vi "配置数据迁移.vi"(8 "error in (no error)":errorcluster) -> (0 "error out":errorcluster)   [LabVIEW 2016]
uses:
  <vilib>/Utility/config.llb/Read Key (String).vi
  <vilib>/Utility/config.llb/Write Key (String).vi
  <vilib>/Utility/config.llb/NI_LVConfig.lvlib
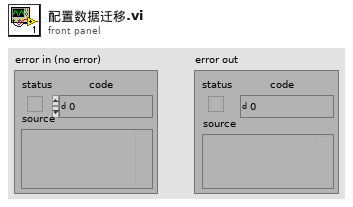
[diagram p1: front panel]
types:
  T1 = typedef "NI_LVConfig.lvlib/Config Data RefNum.ctl" = refnum<k1>
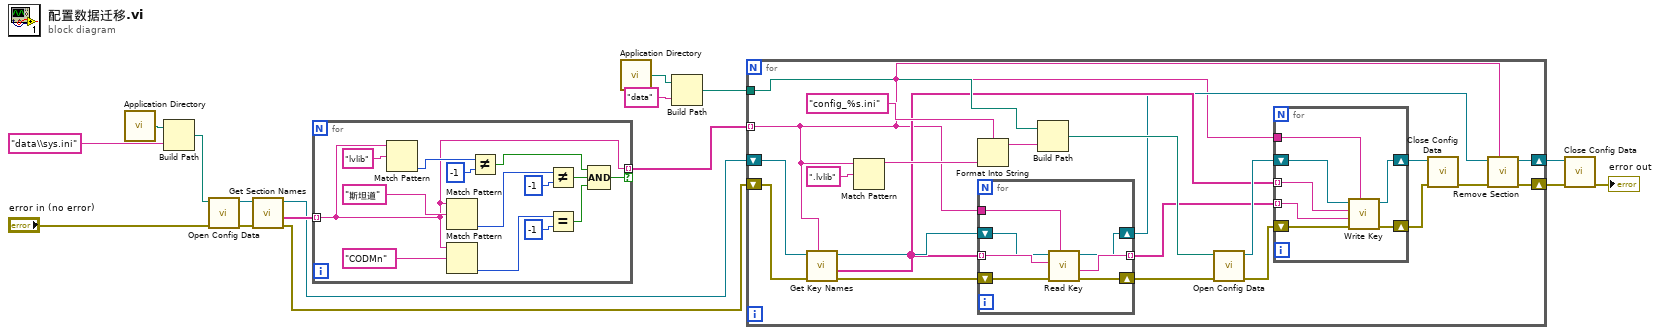
[diagram p0: block diagram]
diagram:
  n1 = call <vilib>:"Application Directory.vi"() -> ("Application Directory"=w14:path)
  n2 = Build Path(base path=w14, name or relative path="data\\sys.ini" ("名称或相对路径")) -> (appended path=w16:path)
  n3 = call <vilib>:"Open Config Data.vi"("error in (no error)"="error in (no error)", "configuration file path"=w16) -> ("error out"=w13:errorcluster, "refnum"=w12:T1)  [unwired: 7 in, 1 out]
  n4 = call <vilib>:"Get Section Names.vi"("error in (no error)"=w13, "refnum"=w12) -> ("error out"=w4:errorcluster, "section names"=w11:string[], "refnum out"=w10:T1)  [unwired: 7 in]
  n5 = for {
    tunnel: w11 -> [w25] mode=indexing
    tunnel: [w25] -> w9 mode=indexing if=w17
    n6 = Match Pattern(string=w25, regular expression="lvlib" ("正则表达式")) -> (offset past match=w29:i32)  [unwired: 1 in, 3 out]
    n7 = Match Pattern(string=w25, regular expression="斯坦道" ("正则表达式")) -> (offset past match=w24:i32)  [unwired: 1 in, 3 out]
    n8 = Match Pattern(string=w25, regular expression="CODMn" ("正则表达式")) -> (offset past match=w23:i32)  [unwired: 1 in, 3 out]
    n9 = Not Equal?(x=w29, y=-1) -> (x != y?=w20:bool)
    n10 = Not Equal?(x=w24, y=-1) -> (x != y?=w19:bool)
    n11 = Equal?(x=w23, y=-1) -> (x = y?=w18:bool)
    n12 = Compound Arithmetic op=AND ("复合运算")(w20, w19, w18) -> (w17:bool)
  }
  n13 = call <vilib>:"Application Directory.vi"() -> ("Application Directory"=w8:path)
  n14 = Build Path(base path=w8, name or relative path="data" ("名称或相对路径")) -> (appended path=w6:path)
  n15 = for {
    tunnel: w9 -> [w34] mode=indexing
    tunnel: w6 -> [w47]
    shift-right: [w33] -> w5
    shift-left: w10 -> [w52]
    shift-right: [w31] -> w3
    shift-left: w4 -> [w32]
    n16 = call <vilib>:"Get Key Names.vi"("section"=w34, "error in (no error)"=w32, "refnum"=w52) -> ("error out"=w51:errorcluster, "key names"=w40:string[], "refnum out"=w50:T1)  [unwired: 5 in, 1 out]
    n17 = Match Pattern(string=w34, regular expression=".lvlib" ("正则表达式")) -> (before substring=w44:string)  [unwired: 1 in, 3 out]
    n18 = Format Into String(format string="config_%s.ini" ("格式字符串"), w44) -> (resulting string=w43:string)  [unwired: 2 in, 1 out]
    n19 = for {
      tunnel: w40 -> [w66] mode=indexing
      tunnel: w34 -> [w65]
      tunnel: [w64] -> w39 mode=indexing
      shift-right: [w62] -> w49
      shift-left: w51 -> [w63]
      shift-right: [w60] -> w35
      shift-left: w50 -> [w61]
      n20 = call-poly <vilib>:"Read Key.vi"("section"=w65, "error in (no error)"=w63, "key"=w66, "refnum"=w61) -> ("error out"=w62:errorcluster, "value"=w64:string, "refnum out"=w60:T1)  [unwired: 4 in, 1 out]
    }
    n21 = Build Path(base path=w47, name or relative path=w43) -> (appended path=w42:path)
    n22 = call <vilib>:"Open Config Data.vi"("error in (no error)"=w49, "configuration file path"=w42) -> ("error out"=w48:errorcluster, "refnum"=w41:T1)  [unwired: 7 in, 1 out]
    n23 = for {
      tunnel: w34 -> [w57]
      tunnel: w40 -> [w56] mode=indexing
      tunnel: w39 -> [w55] mode=indexing
      shift-right: [w54] -> w37
      shift-left: w41 -> [w58]
      shift-right: [w53] -> w38
      shift-left: w48 -> [w59]
      n24 = call-poly <vilib>:"Write Key.vi"("section"=w57, "error in (no error)"=w59, "value"=w55, "key"=w56, "refnum"=w58) -> ("error out"=w53:errorcluster, "refnum out"=w54:T1)  [unwired: 4 in, 1 out]
    }
    n25 = call <vilib>:"Close Config Data.vi"("error in (no error)"=w38, "refnum"=w37) -> ("error out"=w36:errorcluster)  [unwired: 8 in, 1 out]
    n26 = call <vilib>:"Remove Section.vi"("section"=w34, "error in (no error)"=w36, "refnum"=w35) -> ("error out"=w31:errorcluster, "refnum out"=w33:T1)  [unwired: 6 in, 1 out]
  }
  n27 = call <vilib>:"Close Config Data.vi"("error in (no error)"=w3, "refnum"=w5) -> ("error out"=→"error out":errorcluster)  [unwired: 8 in, 1 out]
